vi "Lin_Rohner_lab4A_Compensation_JustG.vi"() -> ()   [LabVIEW 2019]
uses:
  <vilib>/Platform/TimedLoop/XDataNode/timing_clust.ctl
  <vilib>/Platform/TimedLoop/XDataNode/nitl_modes.ctl
  <vilib>/Platform/TimedLoop/XDataNode/wakeup.ctl
  <vilib>/Analysis/3filter.llb/Filter Passband Type.ctl
  <vilib>/DAQmx/write.llb/DAQmx Write (Analog DBL 1Chan 1Samp).vi
  <vilib>/DAQmx/read.llb/DAQmx Read (Analog DBL 1Chan 1Samp).vi
  <vilib>/DAQmx/create/channels.llb/DAQmx Create Channel (AO-Voltage-Basic).vi
  <vilib>/DAQmx/miscellaneous.llb/DAQmx Fill In Error Info.vi
  <vilib>/DAQmx/create/channels.llb/DAQmx Create Channel (AI-Voltage-Basic).vi
  <vilib>/platform/TimedLoop/XDataNode/XDataNode.xnode
  <vilib>/Platform/TimedLoop/XDataNode/XDNodeRunTimeDep.lvlib
  <vilib>/ptbypt/NI_PtbyPt.lvlib
  <vilib>/Analysis/NI_AALBase.lvlib
panel:
  out "Compensation Voltage":dbl
  out "Compensation Voltage":dbl(graph)
  out "Gravity Compesation":dbl
  in  "Gravaty Compensation":bool
  out "Filtered Angular Position [deg]":dbl(graph)
  out "Filtered Angular Position [deg]":dbl
  out "Gravity Compesation":dbl(graph)
  in  "low cutoff freq: Position":dbl=0.125 format="%0.3f"
  in  "stop":bool
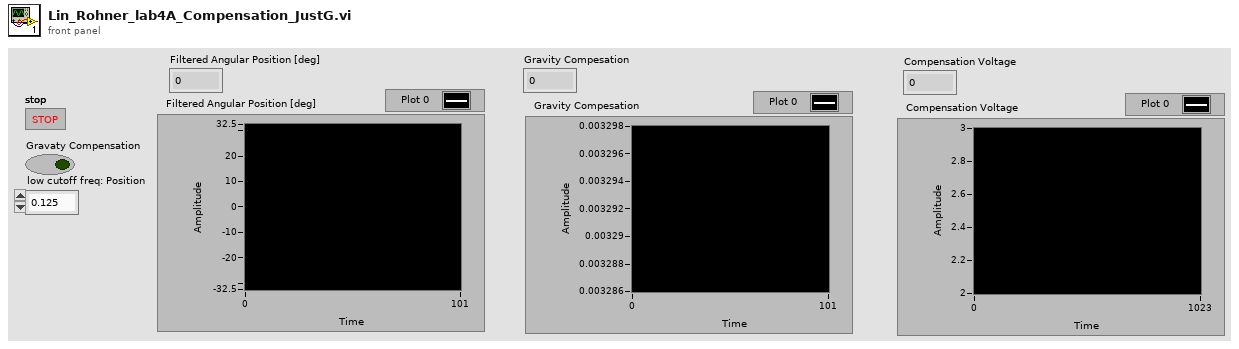
[diagram p1: front panel]
types:
  T1 = typedef "NI_AALBase.lvlib/Filter Passband Type.ctl" = enum32{"Lowpass", "Highpass", "Bandpass", "Bandstop"}
  T2 = typedef "XDNodeRunTimeDep.lvlib/timing_clust.ctl" = cluster{"Expected End [f-1]":u64, "Actual End [f-1]":u64, "Finished Late? [f-1]":bool, "Expected End [i-1]":u64, "Actual End [i-1]":u64, "Finished Late? [i-1]":bool, "Expected Start [i]":u64, "Actual Start [i]":u64, "Expected Start [f]":u64, "Actual Start [f]":u64, "Source Name":string, "Structure Name":string, "Period":i64, "Deadline":i64, "Offset":i64, "Start":i64, "Priority":i32, "Timeout":i32, "Mode":T3, "Wakeup Reason":T4, "Error":errorcluster, "Source Type":string, "Secondary Source Type":string, "Global End Time":u64, "Global Start Time":u64, "Frame Duration":u64, "Iteration Duration":u64, "Assigned CPU":i32, "I/O Scan Engine Mode":u32}
  T3 = typedef "XDNodeRunTimeDep.lvlib/nitl_modes.ctl" = enum32{"No Change", "Process missed periods, maintain original phase", "Discard missed periods, maintain original phase", "Process missed periods, ignore original phase", "Discard missed periods, ignore original phase"}
  T4 = typedef "XDNodeRunTimeDep.lvlib/wakeup.ctl" = enum32{"Normal", "Aborted", "Asynchronous wakeup", "Timing source error", "Timed loop error", "Timeout"}
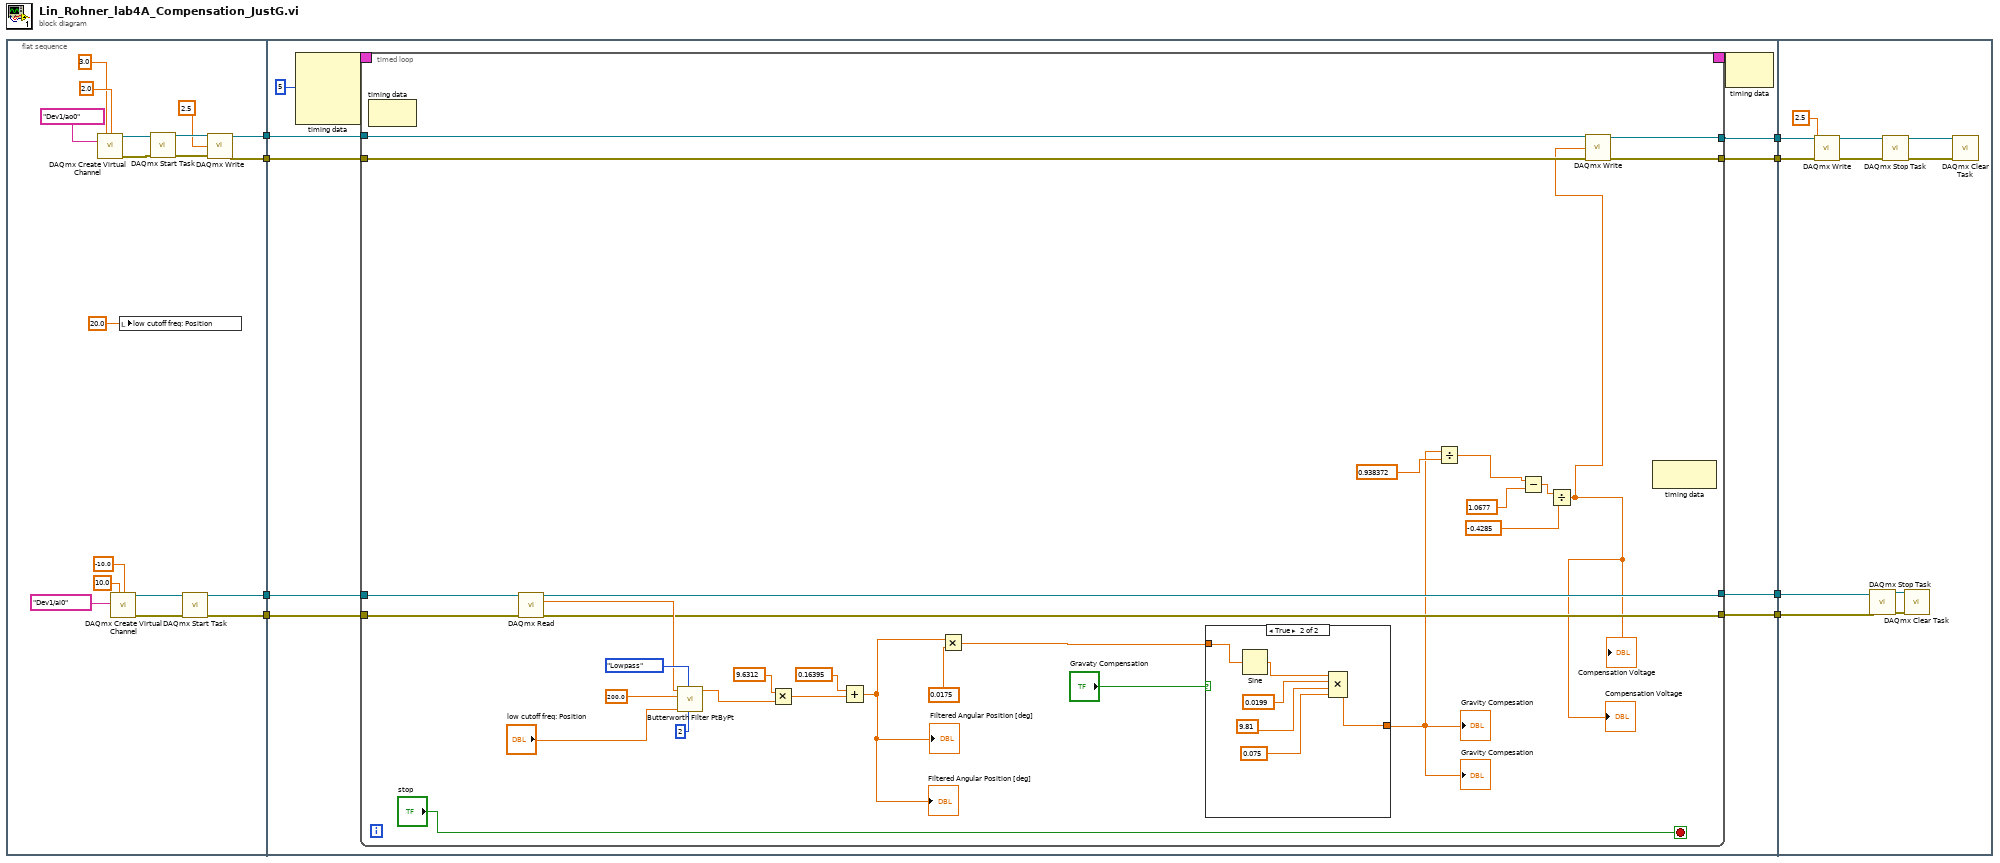
[diagram p0: block diagram]
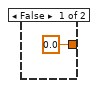
[diagram p2: hidden frame]
diagram:
  n1 = flat-sequence {
    tunnel: [w24] -> w8
    tunnel: [w23] -> w7
    tunnel: [w12] -> w6
    tunnel: [w11] -> w5
    tunnel: w8 -> [w34]
    tunnel: w7 -> [w33]
    tunnel: w6 -> [w32]
    tunnel: w5 -> [w31]
    tunnel: [w30] -> w4
    tunnel: [w29] -> w3
    tunnel: [w28] -> w2
    tunnel: [w27] -> w1
    tunnel: w4 -> [w83]
    tunnel: w3 -> [w82]
    tunnel: w2 -> [w81]
    tunnel: w1 -> [w80]
    frame #0 {
      n2 = call-poly <vilib>:"DAQmx Create Virtual Channel.vi"("maximum value"=3.0, "minimum value"=2.0, "physical channels"=tag "Dev1/ao0") -> ("task out"=w26:refnum<k21>, "error out"=w22:errorcluster)  [unwired: 11 in]
      n3 = call-poly <vilib>:"DAQmx Create Virtual Channel.vi"("maximum value"=10.0, "minimum value"=-10.0, "physical channels"=tag "Dev1/ai0") -> ("task out"=w13:refnum<k21>, "error out"=w14:errorcluster)  [unwired: 11 in]
      n4 = local write "low cutoff freq: Position"(20.0 ("low cutoff freq: Position")) -> ()
      n5 = call <vilib>:"DAQmx Start Task.vi"("task/channels in"=w26, "error in"=w22) -> ("task out"=w25:refnum<k21>, "error out"=w21:errorcluster)  [unwired: 12 in]
      n6 = call <vilib>:"DAQmx Start Task.vi"("task/channels in"=w13, "error in"=w14) -> ("task out"=w12:refnum<k21>, "error out"=w11:errorcluster)  [unwired: 12 in]
      n7 = call-poly <vilib>:"DAQmx Write.vi"("task/channels in"=w25, "data"=2.5, "error in"=w21) -> ("task out"=w24:refnum<k21>, "error out"=w23:errorcluster)  [unwired: 10 in, 1 out]
    }
    frame #1 {
      n8 = node-c288(i64 5 ("Period")) -> (w37:T2)  [unwired: 3 in]
      n9 = timed-loop {
        timing: w37 -> [_]
        timing-out: [_] -> w36
        tunnel: w34 -> [w58]
        tunnel: w33 -> [w57]
        tunnel: w32 -> [w56]
        tunnel: w31 -> [w55]
        tunnel: [w51] -> w30
        tunnel: [w50] -> w29
        tunnel: [w54] -> w28
        tunnel: [w53] -> w27
        stop <- "stop" stop-if-true
        n10 = node-c288() -> ()  [unwired: 1 in, 1 out]
        n11 = call-poly <vilib>:"DAQmx Read.vi"("task/channels in"=w56, "error in"=w55) -> ("task out"=w54:refnum<k21>, "data"=w59:dbl, "error out"=w53:errorcluster)  [unwired: 11 in]
        n12 = call <vilib>:"Butterworth Filter PtByPt.vi"("order"=2, "filter type"=Filter_Passband_Type."Lowpass", "low cutoff freq: fl"="low cutoff freq: Position", "sampling freq: fs"=200.0, "x"=w59) -> ("Filtered x"=w60:dbl)  [unwired: 4 in, 1 out]
        n13 = Multiply(x=9.6312, y=w60) -> (x*y=w62:dbl)
        n14 = Add(x=0.16395, y=w62) -> (x+y=w48:dbl)
        "Filtered Angular Position [deg]" <- w48
        "Filtered Angular Position [deg]" <- w48
        n15 = Multiply(x=w48, y=0.0175) -> (x*y=w46:dbl)
        n16 = case shown="True" "Gravaty Compensation" {
          tunnel: [0.0 w69] -> w38
          tunnel: w46 -> [_ w68]
          frame False {
          }
          frame True {
            n17 = Sine(x=w68) -> (sin(x)=w73:dbl)
            n18 = Compound Arithmetic op=MULTIPLY(w73, 0.0199 ("y"), 9.81 ("value"), 0.075 ("value")) -> (w69:dbl)
          }
        }
        "Gravity Compesation" <- w38
        "Gravity Compesation" <- w38
        n19 = Divide(x=w38, y=0.938372) -> (x/y=w39:dbl)
        n20 = Subtract(x=w39, y=1.0677) -> (x-y=w43:dbl)
        n21 = Divide(x=w43, y=-0.4285) -> (x/y=w41:dbl)
        "Compensation Voltage" <- w41
        "Compensation Voltage" <- w41
        n22 = call-poly <vilib>:"DAQmx Write.vi"("task/channels in"=w58, "data"=w41, "error in"=w57) -> ("task out"=w51:refnum<k21>, "error out"=w50:errorcluster)  [unwired: 10 in, 1 out]
        n23 = node-c288() -> ()  [unwired: 1 in, 1 out]
      }
      n24 = node-c288(w36) -> ()  [unwired: 1 out]
    }
    frame #2 {
      n25 = call-poly <vilib>:"DAQmx Write.vi"("task/channels in"=w83, "data"=2.5, "error in"=w82) -> ("task out"=w90:refnum<k21>, "error out"=w87:errorcluster)  [unwired: 10 in, 1 out]
      n26 = call <vilib>:"DAQmx Stop Task.vi"("task/channels in"=w81, "error in"=w80) -> ("task out"=w84:refnum<k21>, "error out"=w85:errorcluster)  [unwired: 12 in]
      n27 = call <vilib>:"DAQmx Stop Task.vi"("task/channels in"=w90, "error in"=w87) -> ("task out"=w89:refnum<k21>, "error out"=w88:errorcluster)  [unwired: 12 in]
      n28 = call <vilib>:"DAQmx Clear Task.vi"("task in"=w84, "error in"=w85) -> ()  [unwired: 13 in, 1 out]
      n29 = call <vilib>:"DAQmx Clear Task.vi"("task in"=w89, "error in"=w88) -> ()  [unwired: 13 in, 1 out]
    }
  }
